vi "Read Macro Names.vi"(8 "error in (no error)":errorcluster, 11 "Macro Directory":path) -> (0 "error out":errorcluster, 3 "Macro Names":string[](array[string]))   [LabVIEW 2020, in "MacroAssert.lvlib"]
doc: "Reads the list of macro names from <B>App Data Directory</B>."
uses:
  MacroAssert.lvlib
  <userlib>/_OpenG.lib/file/file.llb/openg_file.lvlib
  <userlib>/_OpenG.lib/file/file.llb/Strip Path Extension - 1D Array of Strings__ogtk.vi
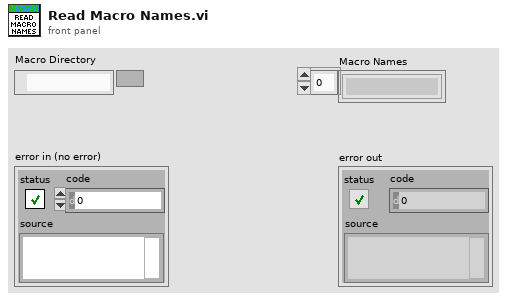
[diagram p1: front panel]
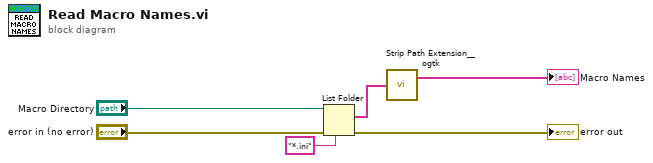
[diagram p0: block diagram]
diagram:
  n1 = List Folder(path="Macro Directory", pattern="*.ini", error in="error in (no error)") -> (filenames=w4:string[], error out=→"error out":errorcluster)  [unwired: 1 in, 2 out]
  n2 = call-poly <userlib>:"Strip Path Extension__ogtk.vi"("paths"=w4) -> ("roots"=→"Macro Names":string[])  [unwired: 1 out]
